vi "cRIO_FPGA_COMMUNICATION Handle FPGA.vi"(8 "error in (no error)":errorcluster caption="Fehler (Eingang, kein Fehler)", 11 "Ressourcenname":T1 caption="RIO Device") -> (0 "error out":errorcluster caption="Fehler (Ausgang)")   [LabVIEW 2013, in "cRIO_FPGA_COMMUNICATION.lvlib"]
uses:
  cRIO_FPGA_COMMUNICATION.lvlib
  <vilib>/userdefined/High Color/nirio_resource_hc.ctl
  TYPES/TYPE FPGA States.ctl
  <vilib>/Platform/TimedLoop/XDataNode/timing_clust.ctl
  <vilib>/Platform/TimedLoop/XDataNode/nitl_modes.ctl
  <vilib>/Platform/TimedLoop/XDataNode/wakeup.ctl
  TYPES/TYPE Band und Stations Kommandos.ctl
  <vilib>/FPGAPlugInAG/cRIO-9114/niLvFpga_Open_cRIO-9114.vi
  <vilib>/Utility/error.llb/Error Cluster From Error Code.vi
  <vilib>/rvi/errors/niLvFpgaAdjustHostInterfaceError.vi
  GLOBALS/cRIO_FPGA_COMMUNICATION Global.vi
  <vilib>/rvi/interface/common/niFpgaWaitOnOcc.vi
  <vilib>/FPGAPlugInAG/cRIO-9114/niLvFpga_Close_cRIO-9114.vi
  <vilib>/Platform/TimedLoop/XDataNode/XDataNode.xnode
  <vilib>/rvi/interface/nirviOpenFPGA/nirviOpenFPGA.xnode
  FPGA Bitfiles/Test_FPGATarget_CScRIOPBFPGADP-M_4E0AD52E.lvbitx
  <vilib>/rvi/interface/nirviReadWriteControl/nirviReadWriteControl.xnode
  <vilib>/rvi/interface/nirviMethod/nirviMethod.xnode
  <vilib>/rvi/interface/nirviCloseFPGA/nirviCloseFPGA.xnode
  <vilib>/Platform/TimedLoop/XDataNode/XDNodeRunTimeDep.lvlib
  <vilib>/FPGAPlugInAG/cRIO-9114/niLvFpga_ReadFifo_cRIO-9114.vi
  <vilib>/rvi/errors/niLvFpgaMergeErrorWithErrorCode.vi
  NiFpgaLv.dll
panel:
  out "Verspätete Beendigung? [i-1]":bool
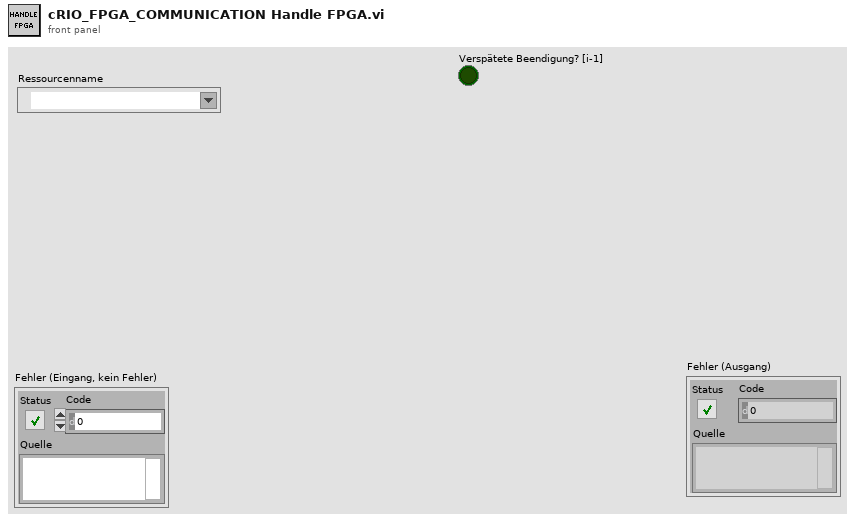
[diagram p1: front panel]
types:
  T1 = typedef "nirio_resource_hc.ctl" = tag
  T2 = typedef "cRIO_FPGA_COMMUNICATION.lvlib/TYPE FPGA States.ctl" = enum16{"Init FPGA/Analysation", "Run FPGA/Analysation", "Deinit FPGA"}
  T3 = enum16{"Init", "Zählerkonfig. setzen", "lese Zählerkonfig."}
  T4 = enum16{"Init", "Zählerwert nullen", "Zählerwert setzen", "lese gesetzten Zählerwert"}
  T5 = enum16{"Init", "Zählerwert updaten", "Zählerwert lesen"}
  T6 = typedef "cRIO_FPGA_COMMUNICATION.lvlib/TYPE Band und Stations Kommandos.ctl" = enum16{"Init", "Lese", "Schreibe"}
  T7 = enum16{"Init", "set Counter", "get Counter", "reset Counter", "configure Counter"}
  T8 = typedef "XDNodeRunTimeDep.lvlib/timing_clust.ctl" = cluster{"Expected End [f-1]":u64, "Actual End [f-1]":u64, "Finished Late? [f-1]":bool, "Expected End [i-1]":u64, "Actual End [i-1]":u64, "Finished Late? [i-1]":bool, "Expected Start [i]":u64, "Actual Start [i]":u64, "Expected Start [f]":u64, "Actual Start [f]":u64, "Source Name":string, "Structure Name":string, "Period":i64, "Deadline":i64, "Offset":i64, "Start":i64, "Priority":i32, "Timeout":i32, "Mode":T9, "Wakeup Reason":T10, "Error":errorcluster, "Source Type":string, "Secondary Source Type":string, "Global End Time":u64, "Global Start Time":u64, "Frame Duration":u64, "Iteration Duration":u64, "Assigned CPU":i32, "I/O Scan Engine Mode":u32}
  T9 = typedef "XDNodeRunTimeDep.lvlib/nitl_modes.ctl" = enum32{"No Change", "Process missed periods, maintain original phase", "Discard missed periods, maintain original phase", "Process missed periods, ignore original phase", "Discard missed periods, ignore original phase"}
  T10 = typedef "XDNodeRunTimeDep.lvlib/wakeup.ctl" = enum32{"Normal", "Aborted", "Asynchronous wakeup", "Timing source error", "Timed loop error", "Timeout"}
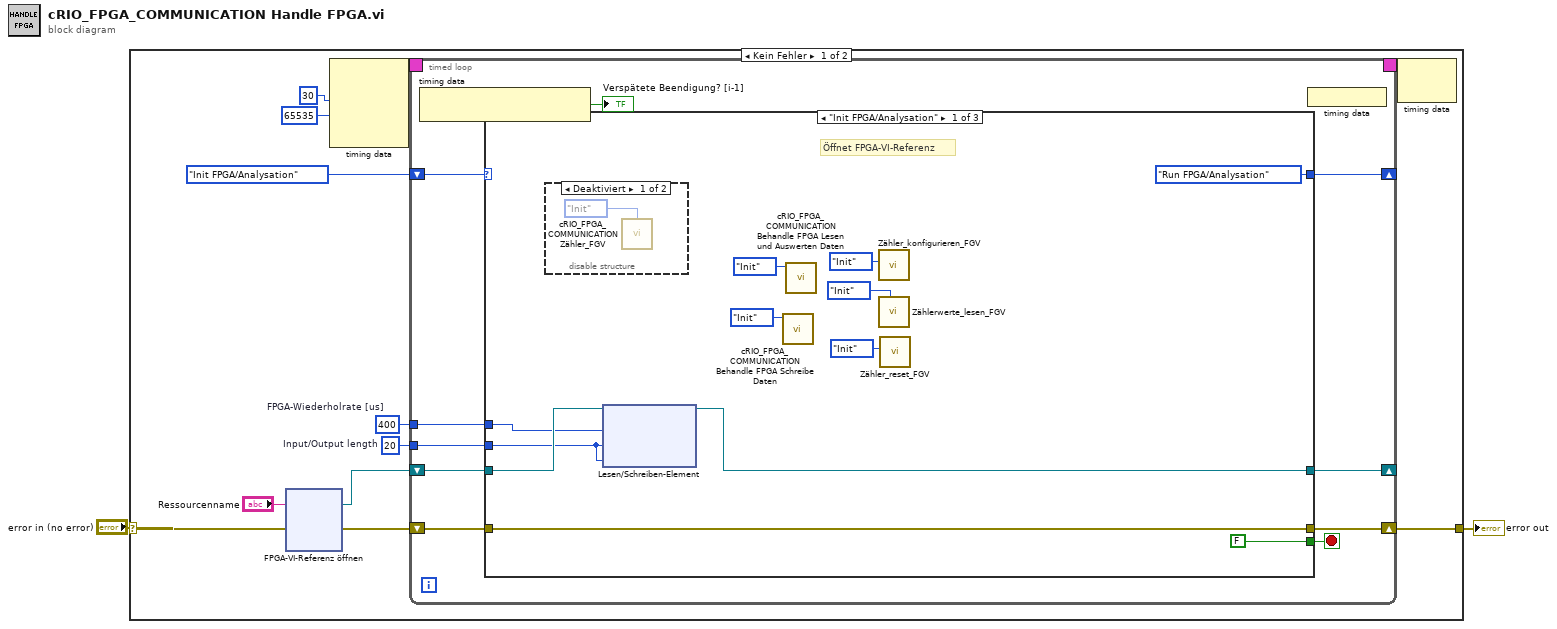
[diagram p0: block diagram]
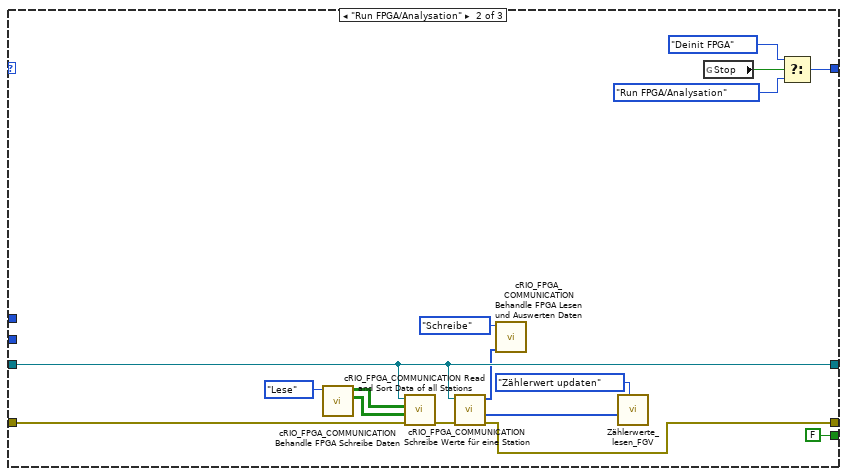
[diagram p3: hidden frame]
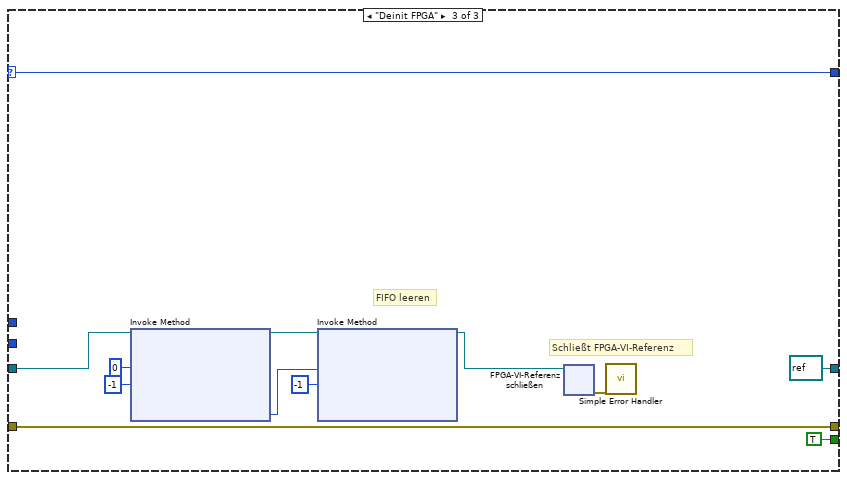
[diagram p4: hidden frame]
diagram:
  n1 = case shown="Kein Fehler" "error in (no error)" {
    selector: "error in (no error)" -> [w7 w74]
    tunnel: [w10 w74] -> w1
    frame No Error {
      w4 = u32 400  # FPGA-Wiederholrate [us]
      w5 = u16 20  # Input/Output length
      n2 = xnode "FPGA-VI-Referenz öffnen"("Fehler (Eingang)"=w7, "Ressourcenname"="Ressourcenname") -> ("FPGA-VI-Referenz (Ausgang)"=w8:refnum<k20>, "Fehler (Ausgang)"=w6:errorcluster)
      n3 = node-c288(i64 30 ("Periode"), 65535 ("Priorität")) -> (w14:T8)  [unwired: 2 in]
      n4 = timed-loop {
        timing: w14 -> [_]
        timing-out: [_] -> w13
        shift-right: [w23] -> _
        shift-left: TYPE_FPGA_States."Init FPGA/Analysation" ("FPGA States") -> [w24]
        shift-right: [w20] -> w10
        shift-left: w6 -> [w19]
        shift-right: [w17] -> _
        shift-left: w8 -> [w22]
        tunnel: w5 -> [w16]
        tunnel: w4 -> [w15]
        stop <- w21 stop-if-true
        n5 = node-c288() -> (→"Verspätete Beendigung? [i-1]":bool)  [unwired: 1 in]
        n6 = case shown="\"Init FPGA/Analysation\"" w24 {
          selector: w24 -> [_ _ w65]
          tunnel: w22 -> [w28 w41 w56]
          tunnel: [TYPE_FPGA_States."Run FPGA/Analysation" ("FPGA States") w51 w65] -> w23
          tunnel: [FALSE FALSE TRUE] -> w21
          tunnel: [w34 w42 w62] -> w20
          tunnel: w19 -> [w34 w43 w62]
          tunnel: [w25 w41 refnum<k20> refnum ("FPGA-VI-Referenz (Ausgang)")] -> w17
          tunnel: w16 -> [w27 _ _]
          tunnel: w15 -> [w26 _ _]
          frame "Init FPGA/Analysation" {
            # "Öffnet FPGA-VI-Referenz"
            n7 = disable-structure shown="Deaktiviert" {
              frame Disabled {
                n8 = call "cRIO_FPGA_COMMUNICATION Zähler_FGV.vi"("Set/Get/Configure"=T7."Init") -> ()  [unwired: 13 in, 2 out]
              }
              frame Enabled {
              }
            }
            n9 = xnode "Lesen/Schreiben-Element"("FPGA-VI-Referenz (Eingang)"=w28, "Delay"=w26, "Output length"=w27, "Input length"=w27) -> ("FPGA-VI-Referenz (Ausgang)"=w25:refnum<k20>)  [unwired: 1 in, 1 out]
            n10 = call "cRIO_FPGA_COMMUNICATION Behandle FPGA Schreibe Daten.vi"("FGV Band/Station Commands"=TYPE_Band_und_Stations_Kommandos."Init") -> ()  [unwired: 9 in, 2 out]
            n11 = call "cRIO_FPGA_COMMUNICATION Behandle FPGA Lesen und Auswerten Daten.vi"("FGV Band/Station Commands"=TYPE_Band_und_Stations_Kommandos."Init") -> ()  [unwired: 10 in, 1 out]
            n12 = call "Zähler_konfigurieren_FGV.vi"("Modus"=T3."Init") -> ()  [unwired: 5 in, 2 out]
            n13 = call "Zählerwerte_lesen_FGV.vi"("Modus"=T5."Init") -> ()  [unwired: 4 in, 3 out]
            n14 = call "Zähler_reset_FGV.vi"("Modus"=T4."Init") -> ()  [unwired: 4 in, 3 out]
          }
          frame "Run FPGA/Analysation" {
            n15 = call "cRIO_FPGA_COMMUNICATION Behandle FPGA Schreibe Daten.vi"("FGV Band/Station Commands"=TYPE_Band_und_Stations_Kommandos."Lese") -> ("Stationen"=w45:bool[][], "Bänder"=w46:bool[][])  [unwired: 9 in]
            n16 = call "cRIO_FPGA_COMMUNICATION  Schreibe Werte für eine Station.vi"("Fehler (Eingang, kein Fehler)"=w43, "Stationen"=w45, "Bänder"=w46, "FPGA-VI-Referenz (Ausgang)"=w41) -> ("Fehler (Ausgang)"=w48:errorcluster)  [unwired: 7 in]
            n17 = call "cRIO_FPGA_COMMUNICATION Read and Sort Data of all Stations.vi"("error in (no error)"=w48, "FPGA-VI-Referenz (Ausgang)"=w41) -> ("error out"=w42:errorcluster, "Zählerwerte (super schneller Counter)"=w39:u16[], "Band & Stationsdaten"=w38:u16[])  [unwired: 7 in]
            n18 = call "cRIO_FPGA_COMMUNICATION Behandle FPGA Lesen und Auswerten Daten.vi"("Band- & Stationsdaten"=w38, "FGV Band/Station Commands"=TYPE_Band_und_Stations_Kommandos."Schreibe") -> ()  [unwired: 9 in, 1 out]
            n19 = call "Zählerwerte_lesen_FGV.vi"("gesammelte Zählerwerte"=w39, "Modus"=T5."Zählerwert updaten") -> ()  [unwired: 3 in, 3 out]
            n20 = global read "cRIO_FPGA_COMMUNICATION Global.vi" "Stop"() -> (w53:bool)
            n21 = Select(t=TYPE_FPGA_States."Deinit FPGA" ("FPGA States"), s=w53, f=TYPE_FPGA_States."Run FPGA/Analysation" ("FPGA States")) -> (s? t:f=w51:T2)
          }
          frame "Deinit FPGA" {
            # "FIFO leeren"
            # "Schließt FPGA-VI-Referenz"
            n22 = xnode "Invoke Method"("FPGA-VI-Referenz (Eingang)"=w56, "Anzahl der Elemente"=u32 0, "Timeout (ms)"=-1) -> ("FPGA-VI-Referenz (Ausgang)"=w55:refnum<k20>, "Verbleibende Elemente"=w60:u32)  [unwired: 1 in, 2 out]
            n23 = xnode "Invoke Method"("FPGA-VI-Referenz (Eingang)"=w55, "Anzahl der Elemente"=w60, "Timeout (ms)"=-1) -> ("FPGA-VI-Referenz (Ausgang)"=w54:refnum<k20>)  [unwired: 1 in, 3 out]
            n24 = xnode "FPGA-VI-Referenz schließen"("FPGA-VI-Referenz (Eingang)"=w54) -> ("Fehler (Ausgang)"=w63:errorcluster)  [unwired: 1 in]
            n25 = call <vilib>:"Simple Error Handler.vi"("error in (no error)"=w63) -> ()  [unwired: 1 in, 8 out]
          }
        }
        n26 = node-c288() -> ()  [unwired: 1 out]
      }
      n27 = node-c288(w13) -> ()  [unwired: 1 out]
    }
    frame Error {
    }
  }
  "error out" <- w1
